vi "modify XML on abort.vi"(11 "frame number":dbl) -> (3 "XML string out":string)   [LabVIEW 2012]
doc: "SciScan 1.2 160622"
uses:
  Custom Controls/scan mode main settings tab.ctl
  GFG/GFGpathGet.vi
  <vilib>/xml/Close Reference(Node).vi
  GFG/GFG library.lvlib
  <resource>/objmgr/DOMUserDefRef.rc
  <vilib>/xml/NI_XML.lvlib
panel:
  out "error out 2":errorcluster
  out "error out":errorcluster
  out "Parse Errors":string
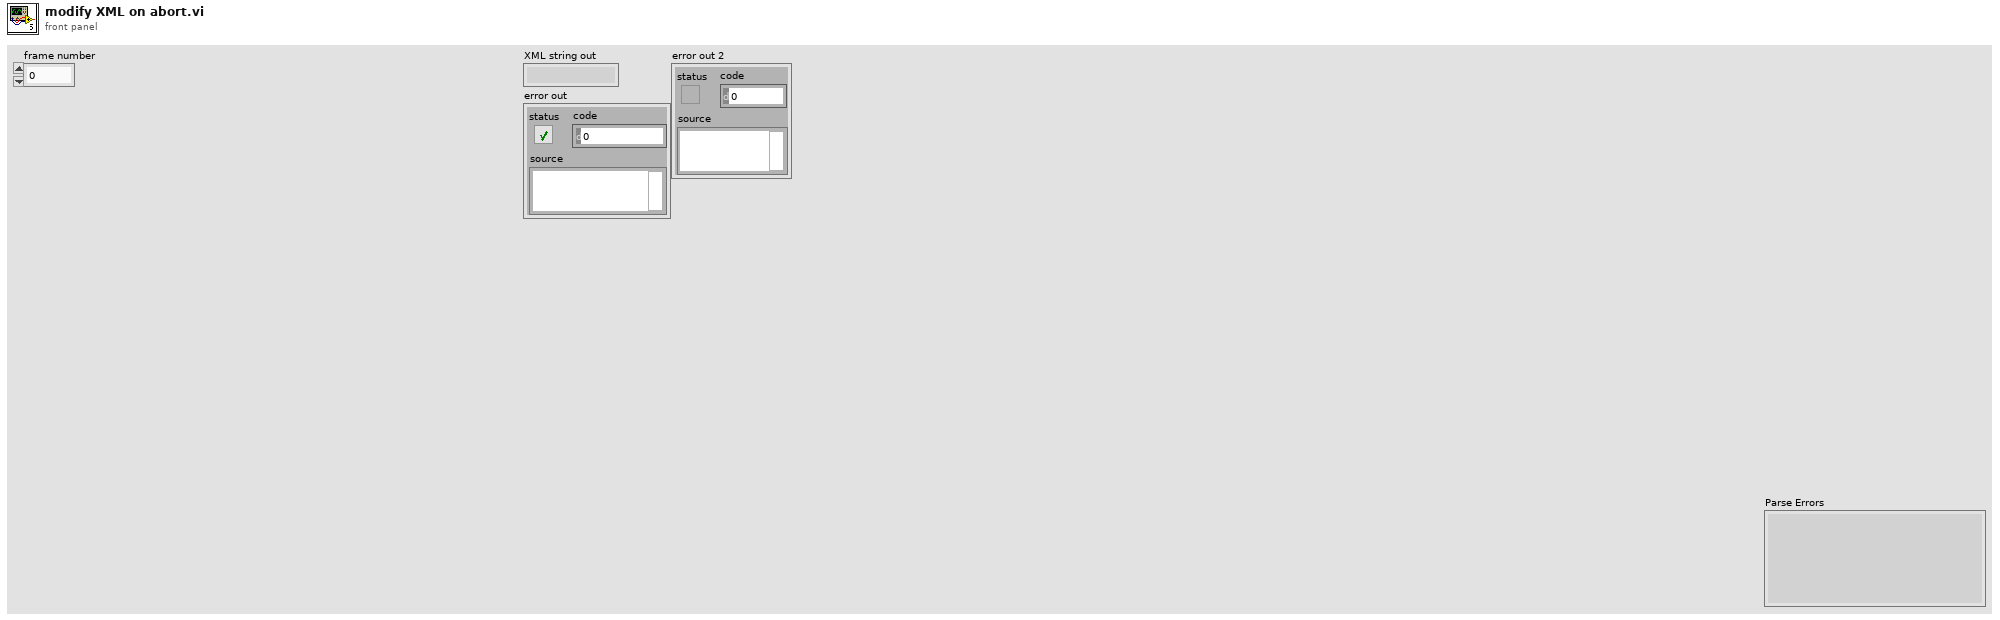
[diagram p1: front panel]
types:
  T1 = typedef "scan mode main settings tab.ctl" = enum32{"2D frame", "2D line scan", "general settings", "Z Stack", "piezo"}
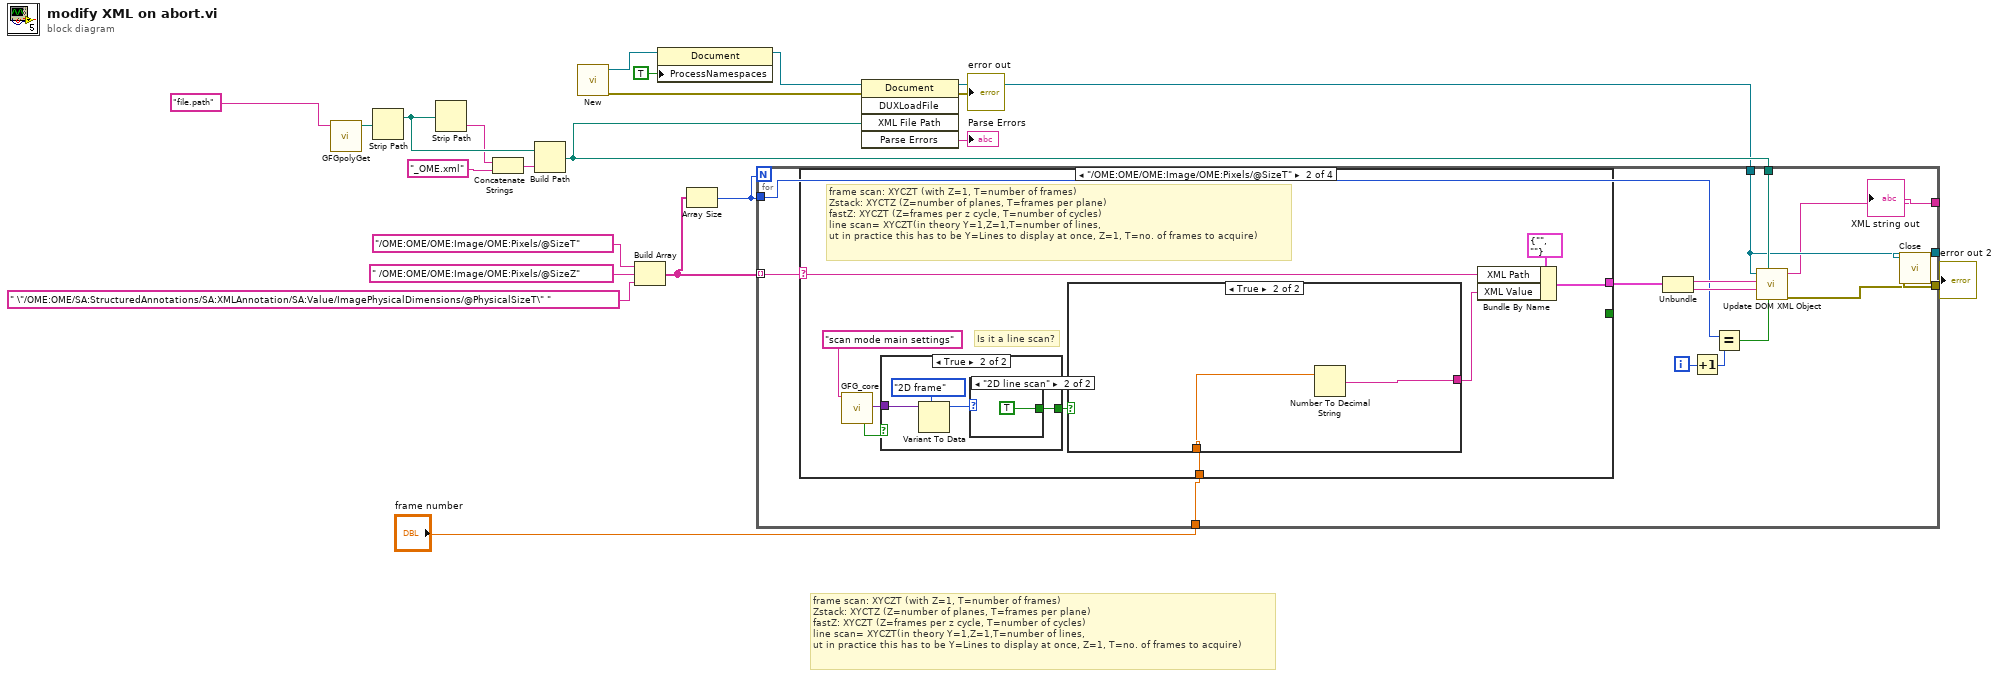
[diagram p0: block diagram]
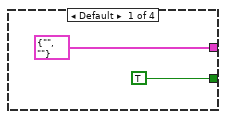
[diagram p2: hidden frame]
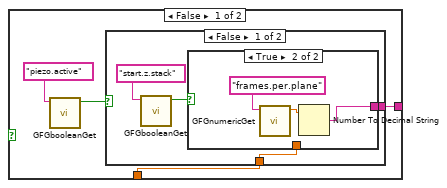
[diagram p3: hidden frame]
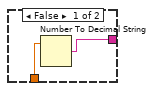
[diagram p4: hidden frame]
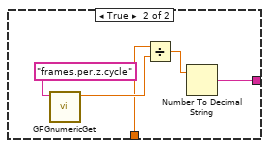
[diagram p5: hidden frame]
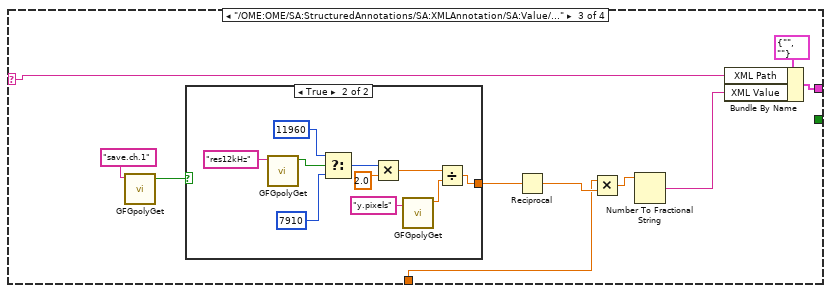
[diagram p8: hidden frame]
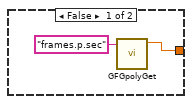
[diagram p9: hidden frame]
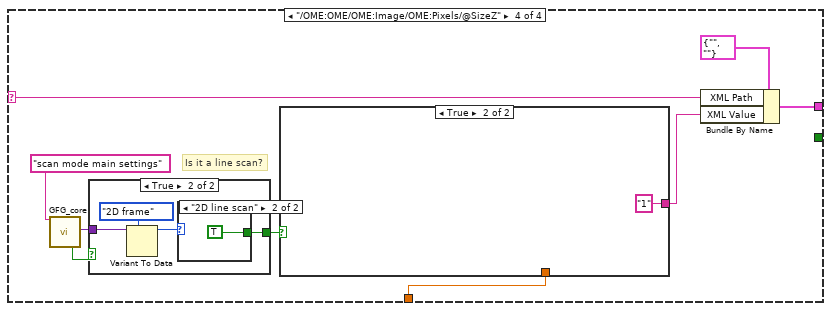
[diagram p10: hidden frame]
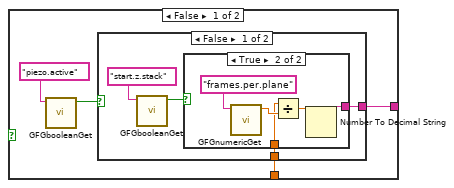
[diagram p11: hidden frame]
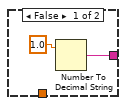
[diagram p12: hidden frame]
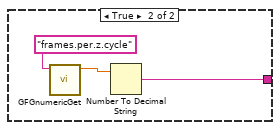
[diagram p13: hidden frame]
diagram:
  # "frame scan: XYCZT (with Z=1, T=number of frames)\nZstack: XYCTZ (Z=number of planes, T=frames per plane)\nfastZ: XYCZT (Z=frames per z cycle, T=number of cycles)\nline scan= XYCZT(in theory Y=1,Z=1,T=number of lines, \nut in practice this has to be Y=Lines to display at once, Z=1, T=no. of frames to acquire)"
  n1 = call-poly "GFGpolyGet.vi"("Variable Name in"="file.path") -> ("Path"=w20:path)  [unwired: 8 in, 2 out]
  n2 = Strip Path(path=w20) -> (stripped path=w19:path)  [unwired: 1 out]
  n3 = Strip Path(path=w19) -> (name=w18:string)  [unwired: 1 out]
  n4 = Concatenate Strings(w18, "_OME.xml" ("string")) -> (w17:string)
  n5 = Build Path(base path=w19, name or relative path=w17) -> (appended path=w10:path)
  n6 = call <vilib>:"New.vi"() -> ("error out"=w15:errorcluster, "DOM document out"=w12:refnum<k20>)  [unwired: 8 in]
  n7 = Build Array("/OME:OME/OME:Image/OME:Pixels/@SizeT", " /OME:OME/OME:Image/OME:Pixels/@SizeZ", " \"/OME:OME/SA:StructuredAnnotations/SA:XMLAnnotation/SA:Value/ImagePhysicalDimensions/@PhysicalSizeT\" ") -> (w2:string[])
  n8 = property class="Document"(reference=w12, "ProcessNamespaces"=TRUE ("Process Namespaces")) -> (reference out=w11:refnum<k20>)  [unwired: 1 in, 1 out]
  n9 = Array Size(array=w2) -> (size(s)=w1:i32)
  n10 = invoke class="Document" method="DUXLoadFile"(reference=w11, error in=w15, "XML File Path"=w10) -> (reference out=w9:refnum<k20>, error out=→"error out":errorcluster, "Parse Errors"=→"Parse Errors":string)  [unwired: 2 in, 2 out]
  n11 = for {
    N: w1 -> [_]
    tunnel: w2 -> [w37] mode=indexing
    tunnel: "frame number" -> [w36]
    tunnel: w9 -> [w29]
    tunnel: w10 -> [w31]
    tunnel: [w30] -> w8
    tunnel: [w29] -> w7
    tunnel: [w28] -> w6
    tunnel: w1 -> [w26]
    i -> [w27]
    n12 = case shown="\"/OME:OME/OME:Image/OME:Pixels/@SizeT\"" w37 {
      selector: w37 -> [_ w46 w75 w104]
      tunnel: [cluster{"XML Path":string, "XML Value":string} {"XML Path"="", "XML Value"=""} ("Path-Value pairs") w47 w76 w97] -> w35
      tunnel: [TRUE _ _ _] -> _
      tunnel: w36 -> [_ w40 w74 w96]
      frame Default {
      }
      frame "/OME:OME/OME:Image/OME:Pixels/@SizeT" {
        # "frame scan: XYCZT (with Z=1, T=number of frames)\nZstack: XYCTZ (Z=number of planes, T=frames per plane)\nfastZ: XYCZT (Z=frames per z cycle, T=number of cycles)\nline scan= XYCZT(in theory Y=1,Z=1,T=number of lines, \nut in practice this has to be Y=Lines to display at once, Z=1, T=no. of frames to acquire)"
        # "Is it a line scan?"
        n13 = call "GFG_core.vi"("Variable Name in"="scan mode main settings") -> ("Found/Replaced"=w45:bool, "Variant Out"=w44:variant)  [unwired: 12 in, 5 out]
        n14 = case shown="True" w45 {
          tunnel: w44 -> [_ w72]
          tunnel: [_ w69] -> w42
          frame False {
          }
          frame True {
            n15 = Variant To Data(type=scan_mode_main_settings_tab."2D frame" ("scan mode main settings"), Variant=w72) -> (data=w70:T1)  [unwired: 1 in, 1 out]
            n16 = case shown="\"2D line scan\"" w70 {
              tunnel: [_ TRUE] -> w69
              frame Default {
              }
              frame "2D line scan" {
              }
            }
          }
        }
        n17 = case shown="True" w42 {
          tunnel: [w50 w68] -> w41
          tunnel: w40 -> [w49 w67]
          frame False {
            n18 = call "GFGbooleanGet.vi"("Variable Name in"="piezo.active") -> ("Boolean Value OUT"=w51:bool)  [unwired: 9 in, 1 out]
            n19 = case shown="False" w51 {
              tunnel: [w54 w66] -> w50
              tunnel: w49 -> [w53 w63]
              frame False {
                n20 = call "GFGbooleanGet.vi"("Variable Name in"="start.z.stack") -> ("Boolean Value OUT"=w55:bool)  [unwired: 9 in, 1 out]
                n21 = case shown="True" w55 {
                  tunnel: [w58 w59] -> w54
                  tunnel: w53 -> [w57 _]
                  frame False {
                    n22 = Number To Decimal String(number=w57) -> (decimal integer string=w58:string)  [unwired: 1 in]
                  }
                  frame True {
                    n23 = call "GFGnumericGet.vi"("Variable Name in"="frames.per.plane") -> ("Numeric"=w60:dbl)  [unwired: 8 in, 2 out]
                    n24 = Number To Decimal String(number=w60) -> (decimal integer string=w59:string)  [unwired: 1 in]
                  }
                }
              }
              frame True {
                n25 = call "GFGnumericGet.vi"("Variable Name in"="frames.per.z.cycle") -> ("Numeric"=w64:dbl)  [unwired: 8 in, 2 out]
                n26 = Divide(x=w63, y=w64) -> (x/y=w62:dbl)
                n27 = Number To Decimal String(number=w62) -> (decimal integer string=w66:string)  [unwired: 1 in]
              }
            }
          }
          frame True {
            n28 = Number To Decimal String(number=w67) -> (decimal integer string=w68:string)  [unwired: 1 in]
          }
        }
        n29 = Bundle By Name(cluster=cluster{"XML Path":string, "XML Value":string} {"XML Path"="", "XML Value"=""} ("Path-Value pairs"), "XML Path"=w46, "XML Value"=w41) -> (w47:cluster{"XML Path":string, "XML Value":string})
      }
      frame "/OME:OME/SA:StructuredAnnotations/SA:XMLAnnotation/SA:Value/ImagePhysicalDimensions/@PhysicalSizeT" {
        n30 = call-poly "GFGpolyGet.vi"("Variable Name in"="save.ch.1") -> ("Boolean Value OUT"=w79:bool)  [unwired: 9 in, 1 out]
        n31 = case shown="True" w79 {
          tunnel: [w84 w86] -> w81
          frame False {
            n32 = call-poly "GFGpolyGet.vi"("Variable Name in"="frames.p.sec") -> ("Numeric"=w84:dbl)  [unwired: 8 in, 2 out]
          }
          frame True {
            n33 = call-poly "GFGpolyGet.vi"("Variable Name in"="res12kHz") -> ("Boolean Value OUT"=w93:bool)  [unwired: 9 in, 1 out]
            n34 = Select(t=11960, s=w93, f=7910) -> (s? t:f=w91:i32)
            n35 = Multiply(x=w91, y=2.0) -> (x*y=w88:dbl)
            n36 = call-poly "GFGpolyGet.vi"("Variable Name in"="y.pixels") -> ("Numeric"=w95:dbl)  [unwired: 8 in, 2 out]
            n37 = Divide(x=w88, y=w95) -> (x/y=w86:dbl)
          }
        }
        n38 = Reciprocal(x=w81) -> (1/x=w80:dbl)
        n39 = Multiply(x=w74, y=w80) -> (x*y=w78:dbl)
        n40 = Number To Fractional String(number=w78) -> (F-format string=w77:string)  [unwired: 3 in]
        n41 = Bundle By Name(cluster=cluster{"XML Path":string, "XML Value":string} {"XML Path"="", "XML Value"=""} ("Path-Value pairs"), "XML Path"=w75, "XML Value"=w77) -> (w76:cluster{"XML Path":string, "XML Value":string})
      }
      frame "/OME:OME/OME:Image/OME:Pixels/@SizeZ" {
        # "Is it a line scan?"
        n42 = call "GFG_core.vi"("Variable Name in"="scan mode main settings") -> ("Found/Replaced"=w103:bool, "Variant Out"=w102:variant)  [unwired: 12 in, 5 out]
        n43 = case shown="True" w103 {
          tunnel: w102 -> [_ w127]
          tunnel: [_ w124] -> w100
          frame False {
          }
          frame True {
            n44 = Variant To Data(type=scan_mode_main_settings_tab."2D frame" ("scan mode main settings"), Variant=w127) -> (data=w125:T1)  [unwired: 1 in, 1 out]
            n45 = case shown="\"2D line scan\"" w125 {
              tunnel: [_ TRUE] -> w124
              frame Default {
              }
              frame "2D line scan" {
              }
            }
          }
        }
        n46 = case shown="True" w100 {
          tunnel: [w106 "1"] -> w99
          tunnel: w96 -> [w105 _]
          frame False {
            n47 = call "GFGbooleanGet.vi"("Variable Name in"="piezo.active") -> ("Boolean Value OUT"=w107:bool)  [unwired: 9 in, 1 out]
            n48 = case shown="False" w107 {
              tunnel: [w110 w120] -> w106
              tunnel: w105 -> [w109 _]
              frame False {
                n49 = call "GFGbooleanGet.vi"("Variable Name in"="start.z.stack") -> ("Boolean Value OUT"=w111:bool)  [unwired: 9 in, 1 out]
                n50 = case shown="True" w111 {
                  tunnel: [w114 w116] -> w110
                  tunnel: w109 -> [_ w117]
                  frame False {
                    n51 = Number To Decimal String(number=1.0) -> (decimal integer string=w114:string)  [unwired: 1 in]
                  }
                  frame True {
                    n52 = call "GFGnumericGet.vi"("Variable Name in"="frames.per.plane") -> ("Numeric"=w118:dbl)  [unwired: 8 in, 2 out]
                    n53 = Divide(x=w117, y=w118) -> (x/y=w115:dbl)
                    n54 = Number To Decimal String(number=w115) -> (decimal integer string=w116:string)  [unwired: 1 in]
                  }
                }
              }
              frame True {
                n55 = call "GFGnumericGet.vi"("Variable Name in"="frames.per.z.cycle") -> ("Numeric"=w121:dbl)  [unwired: 8 in, 2 out]
                n56 = Number To Decimal String(number=w121) -> (decimal integer string=w120:string)  [unwired: 1 in]
              }
            }
          }
          frame True {
          }
        }
        n57 = Bundle By Name(cluster=cluster{"XML Path":string, "XML Value":string} {"XML Path"="", "XML Value"=""} ("Path-Value pairs"), "XML Path"=w104, "XML Value"=w99) -> (w97:cluster{"XML Path":string, "XML Value":string})
      }
    }
    n58 = Unbundle(w35) -> ("XML Path"=w34:string, "XML Value"=w33:string)
    n59 = Increment(x=w27) -> (x+1=w25:i32)
    n60 = Equal?(x=w26, y=w25) -> (x = y?=w32:bool)
    n61 = call "Update DOM XML Object.vi"("Write to File?"=w32, "XML File Path"=w31, "New Value (String)"=w33, "XPath expression to node"=w34, "DOM Refnum (XML Document)"=w29) -> ("error out"=w30:errorcluster, "XML string out"=w28:string)  [unwired: 5 in]
  }
  "XML string out" <- w6
  n62 = call-poly <vilib>:"Close.vi"("error in (no error)"=w8, "node"=w7) -> ("error out"=→"error out 2":errorcluster)  [unwired: 7 in]
